vi "Close.vi"(8 "error in (no error)":errorcluster, 11 "ADOResult in":refnum<class "ADOResult.lvclass">) -> (0 "error out":errorcluster)   [LabVIEW 2020, in "ORM_ADONet.lvlib" / "ADOResult.lvclass"]
uses:
  ADOResult.lvclass
  ADOResult.lvclass/ADOResult.ctl
  System.Data
  Read Reader.vi
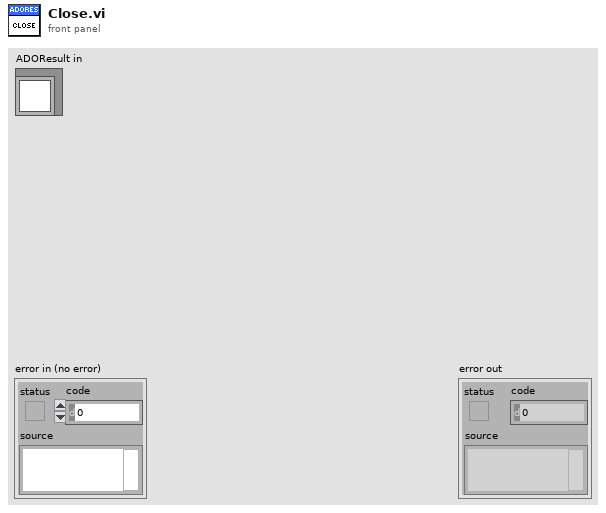
[diagram p1: front panel]
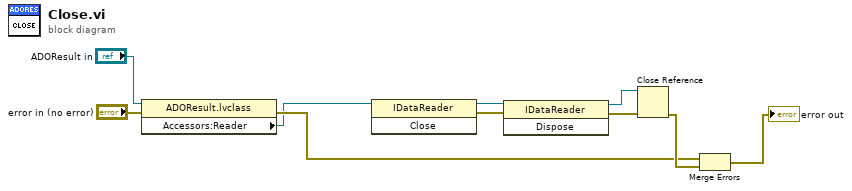
[diagram p0: block diagram]
diagram:
  n1 = property class="ADOResult.lvclass"(reference="ADOResult in", error in="error in (no error)") -> (error out=w3:errorcluster, "Accessors:Reader"=w1:refnum<k24>)  [unwired: 1 out]
  n2 = invoke class="IDataReader" method="Close"(reference=w1) -> (reference out=w10:refnum<k24>, error out=w9:errorcluster)  [unwired: 2 in, 1 out]
  n3 = invoke class="IDataReader" method="Dispose"(reference=w10, error in=w9) -> (reference out=w7:refnum<k24>, error out=w8:errorcluster)  [unwired: 1 in, 1 out]
  n4 = Close Reference(reference=w7, error in (no error)=w8) -> (error out=w5:errorcluster)
  n5 = Merge Errors(w3, w5) -> (→"error out":errorcluster)
